vi "Set or Clear value.vi"(2 "Set clear":T3 {"target value" format="%.1p"}, 3 "Index":u32) -> ()   [LabVIEW 2012]
uses:
  TCP DAQ/Set.ctl
  TCP DAQ/clear offset.ctl
  DAQ configuration/Sensor buffer command.ctl
  global scale array.vi
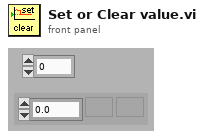
[diagram p1: front panel]
types:
  T1 = typedef "Set.ctl" = bool
  T2 = typedef "clear offset.ctl" = bool
  T3 = cluster{"Set":T1, "target value":dbl, "Clear":T2}
  T4 = typedef "calib array.ctl" = T5[]
  T5 = typedef "conversion.ctl" = cluster{"conversion matrix":sgl[][], "units":string, "name":string, "scale type":T6, "offset (volts)":dbl, "second channel":i8, "correspondence table":T7, "offset (physical units)":dbl, "pH scale":T8, "D.O.":T9}
  T6 = typedef "scale type.ctl" = enum16{"Volts", "Polynomial", "Correspondence Table", "pH", "Dissolved Oxygen", "Quadratic"}
  T7 = typedef "correspondence table.ctl" = cluster{"physical units":dbl, "volts":dbl}[]
  T8 = typedef "pH scale.ctl" = cluster{"Buffers":cluster{"Buffer":dbl, "Calibrated":bool, "V/T":dbl}[], "Temperature":dbl}
  T9 = typedef "DO scale.ctl" = cluster{"Temperature":dbl, "K":dbl, "barometric pressure":dbl}
  T10 = typedef "Sensor buffer command.ctl" = enum16{"read average", "read recent", "read all", "write", "configure", "clear"}
  T11 = typedef "Sensor data.ctl" = cluster{" Sensor array":T12[], "Time":dbl}
  T12 = typedef "sensor cluster.ctl" = cluster{"voltage":sgl, "scaled":sgl, "units":string, "Out of Range":bool}
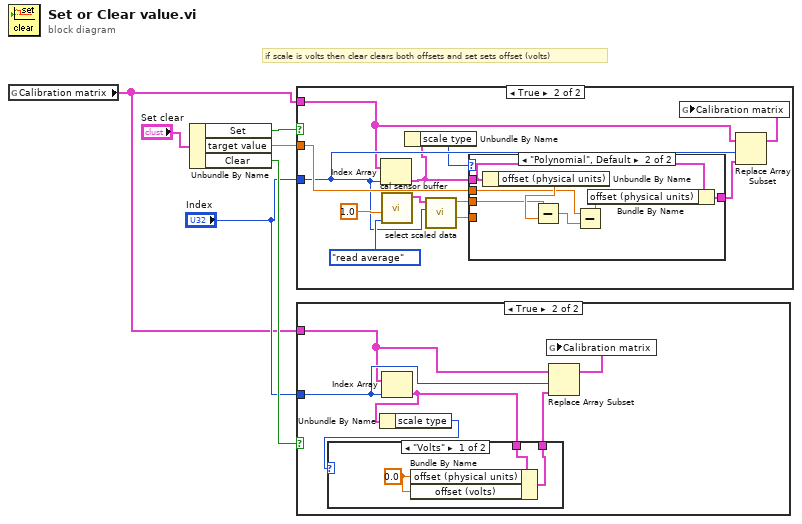
[diagram p0: block diagram]
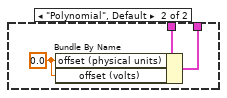
[diagram p3: hidden frame]
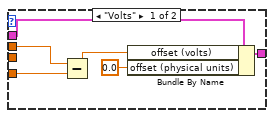
[diagram p5: hidden frame]
diagram:
  # "if scale is volts then clear clears both offsets and set sets offset (volts)"
  n1 = global read "global scale array.vi" "Calibration matrix"() -> (w2:T4)
  n2 = Unbundle By Name("Set clear") -> ("Set"=w5:T1, "target value"=w1:dbl, "Clear"=w4:T2)
  n3 = case shown="True" w5 {
    tunnel: "Index" -> [_ w12]
    tunnel: w2 -> [_ w11]
    tunnel: w1 -> [_ w14]
    frame False {
    }
    frame True {
      n4 = Index Array(array=w11, index=w12) -> (element=w9:T5)
      n5 = call "cal sensor buffer.vi"("command"=Sensor_buffer_command."read average", "smooth interval (s)"=sgl 1.0) -> ("Sensor Data smoothed"=w17:T11)  [unwired: 3 in, 2 out]
      n6 = Unbundle By Name(w9) -> ("scale type"=w8:T6)
      n7 = call "select scaled data.vi"("Sensor index"=w12, "Sensor Data"=w17) -> ("voltage"=w7:sgl, "scaled"=w15:sgl)  [unwired: 4 in, 4 out]
      n8 = case shown="\"Polynomial\", Default" w8 {
        tunnel: w15 -> [_ w27]
        tunnel: w14 -> [w20 w26]
        tunnel: [w24 w31] -> w10
        tunnel: w9 -> [w22 w29]
        tunnel: w7 -> [w19 _]
        frame "Volts" {
          n9 = Subtract(x=w20, y=w19) -> (x-y=w23:dbl)
          n10 = Bundle By Name(cluster=w22, "offset (volts)"=w23, "offset (physical units)"=0.0) -> (w24:T5)
        }
        frame "Polynomial", Default {
          n11 = Unbundle By Name(w29) -> ("offset (physical units)"=w28:dbl)
          n12 = Subtract(x=w27, y=w28) -> (x-y=w25:dbl)
          n13 = Subtract(x=w26, y=w25) -> (x-y=w30:dbl)
          n14 = Bundle By Name(cluster=w29, "offset (physical units)"=w30) -> (w31:T5)
        }
      }
      n15 = Replace Array Subset(array=w11, new element=w10, index=w12) -> (w13:T4)
      n16 = global write "global scale array.vi" "Calibration matrix"(w13) -> ()
    }
  }
  n17 = case shown="True" w4 {
    tunnel: "Index" -> [_ w35]
    tunnel: w2 -> [_ w34]
    frame False {
    }
    frame True {
      n18 = Index Array(array=w34, index=w35) -> (element=w33:T5)
      n19 = Unbundle By Name(w33) -> ("scale type"=w32:T6)
      n20 = case shown="\"Volts\"" w32 {
        tunnel: w33 -> [w40 w43]
        tunnel: [w39 w42] -> w36
        frame "Volts" {
          w38 = 0.0 ("offset (physical units)")
          n21 = Bundle By Name(cluster=w40, "offset (physical units)"=w38, "offset (volts)"=w38) -> (w39:T5)
        }
        frame "Polynomial", Default {
          w41 = 0.0 ("offset (physical units)")
          n22 = Bundle By Name(cluster=w43, "offset (physical units)"=w41, "offset (volts)"=w41) -> (w42:T5)
        }
      }
      n23 = Replace Array Subset(array=w34, new element=w36, index=w35) -> (w37:T4)
      n24 = global write "global scale array.vi" "Calibration matrix"(w37) -> ()
    }
  }
